vi "Update Drawing.vi"(11 "Game Board in":refnum<class "Game Board.lvclass">) -> ()   [LabVIEW 2021, in "Game Board.lvclass"]
doc: "MIT Licence\nCopyright (c) 2024 David Grollier"
uses:
  Game Board.lvclass
  Game Board.lvclass/Game Board.ctl
  Game Board Component/Movable/Movable.lvclass
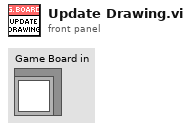
[diagram p1: front panel]
types:
  T1 = map{string, refnum<class "Game Board Component.lvclass">}
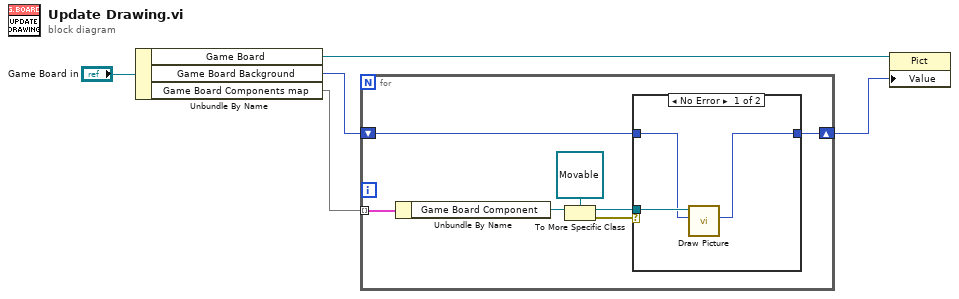
[diagram p0: block diagram]
diagram:
  n1 = Unbundle By Name("Game Board in") -> ("Game Board"=w3:refnum<vi>, "Game Board Background"=w4:picture, "Game Board Components map"=w1:T1)
  n2 = for {
    shift-right: [w7] -> w2
    shift-left: w4 -> [w8]
    tunnel: w1 -> [w10] mode=indexing
    n3 = Unbundle By Name(w10) -> ("Game Board Component"=w11:refnum<class "Game Board Component.lvclass">)
    n4 = To More Specific Class(target class=refnum<class "Movable.lvclass"> refnum ("Movable in"), reference=w11) -> (specific class reference=w9:refnum<class "Movable.lvclass">, error out=w6:errorcluster)  [unwired: 1 in]
    n5 = case shown="No Error" w6 {
      tunnel: w9 -> [w15 _]
      tunnel: w8 -> [w14 w16]
      tunnel: [w13 w16] -> w7
      frame No Error {
        n6 = call-dynamic "Draw Picture.vi"("picture in"=w14, "Movable in"=w15) -> ("picture out"=w13:picture)  [unwired: 9 in]
      }
      frame Error {
      }
    }
  }
  n7 = property class="Pict"(reference=w3, "Value"=w2) -> ()  [unwired: 1 in, 2 out]
